vi "remove_instance.vi"(6 "id (unnamed)":string, 8 "error in (no error)":errorcluster, 9 "Object Instance":refnum<data-value>, 10 "Base Class (LabVIEW Object)":refnum<class>, 11 "Mapped Lookup in":refnum<class "Mapped Lookup.lvclass">) -> (0 "error out":errorcluster, 1 "removed?":bool, 3 "Mapped Lookup out":refnum<class "Mapped Lookup.lvclass">)   [LabVIEW 2019, in "Lookup API.lvlib" / "Mapped Lookup.lvclass"]
uses:
  Mapped Lookup.lvclass
  Mapped Lookup.lvclass/Mapped Lookup.ctl
  <vilib>/Utility/miscctls.llb/LVMapReplaceAction.ctl
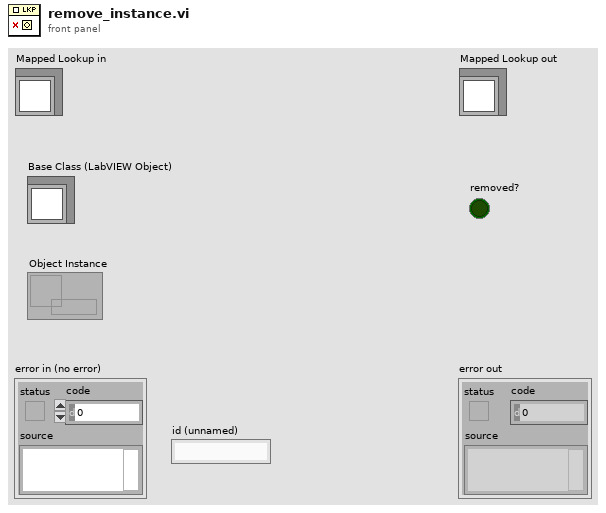
[diagram p1: front panel]
types:
  T1 = typedef "LVMapReplaceAction.ctl" = enum32{"Modify Entry only if found", "Add or Modify Entry", "Delete Entry"}
  T2 = map{string, cluster{"instances":refnum<data-value>, "events":refnum<data-value>}}
  T3 = cluster{"instances":refnum<data-value>, "events":refnum<data-value>}
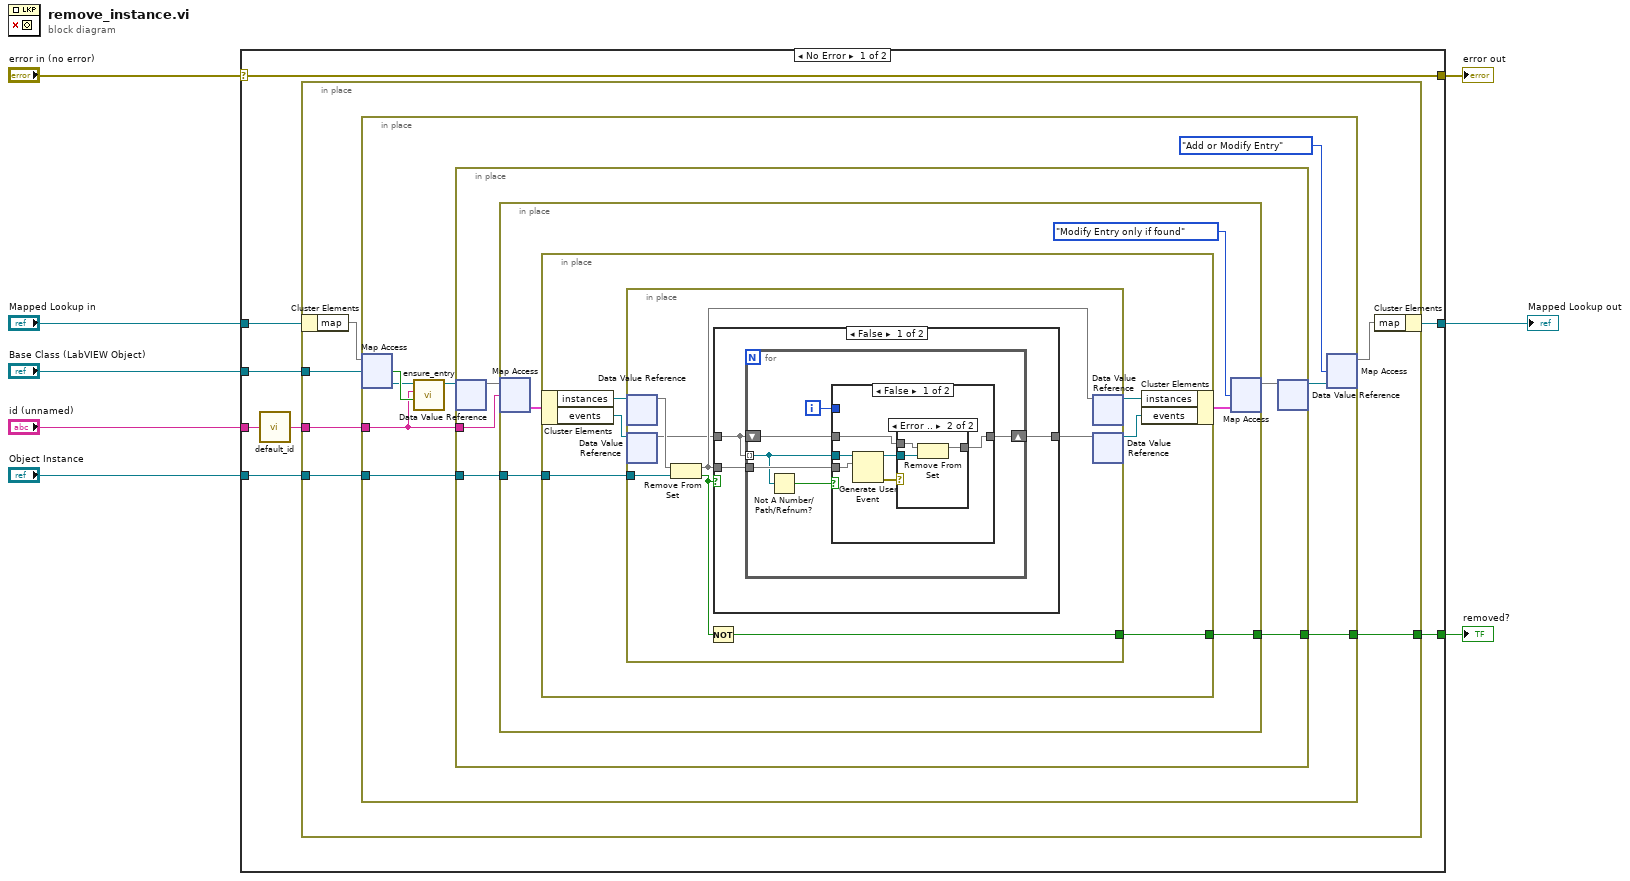
[diagram p0: block diagram]
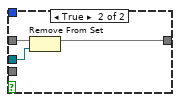
[diagram p3: hidden frame]
diagram:
  n1 = case shown="No Error" "error in (no error)" {
    selector: "error in (no error)" -> [w16 w78]
    tunnel: [w16 w78] -> w5
    tunnel: [w10 w77] -> w6
    tunnel: "Mapped Lookup in" -> [w15 w77]
    tunnel: "Base Class (LabVIEW Object)" -> [w14 _]
    tunnel: "id (unnamed)" -> [w13 _]
    tunnel: "Object Instance" -> [w11 _]
    tunnel: [w9 _] -> w2
    frame No Error {
      n2 = call "default_id.vi"("id (unnamed)"=w13) -> ("String"=w12:string)
      n3 = in-place {
        in-place-border: w14 -> [w18]
        in-place-border: w12 -> [w22]
        in-place-border: w11 -> [w21]
        in-place-border: [w17] -> w9
        n4 = in-place-cluster #1(w15) -> ("map"=w20:map{refnum<class>, refnum<data-value>})
        n5 = in-place {
          in-place-border: w22 -> [w25]
          in-place-border: w21 -> [w28]
          in-place-border: [w23] -> w17
          n6 = in-place-map #2(w20, w18) -> (w27:refnum<data-value>, w29:bool)  [unwired: 1 in]
          n7 = call "ensure_entry.vi"("not found?"=w29, "id"=w25, "named entries in"=w27) -> ("named entries out"=w26:refnum<data-value>)  [unwired: 8 in]
          n8 = in-place {
            in-place-border: w28 -> [w35]
            in-place-border: w25 -> [w33]
            in-place-border: [w31] -> w23
            n9 = in-place-dvr #3(w26) -> (w34:T2)  [unwired: 1 out]
            n10 = in-place {
              in-place-border: w35 -> [w40]
              in-place-border: [w36] -> w31
              n11 = in-place-map #4(w34, w33) -> (w39:T3)  [unwired: 1 in, 1 out]
              n12 = in-place {
                in-place-border: w40 -> [w46]
                in-place-border: [w41] -> w36
                n13 = in-place-cluster #5(w39) -> ("instances"=w45:refnum<data-value>, "events"=w43:refnum<data-value>)
                n14 = in-place {
                  in-place-border: w46 -> [w52]
                  in-place-border: [w48] -> w41
                  n15 = in-place-dvr #6(w45) -> (w53:set{refnum<data-value>})  [unwired: 1 out]
                  n16 = in-place-dvr #7(w43) -> (w50:set{refnum<user-event>})  [unwired: 1 out]
                  n17 = Remove From Set(10:w52, 11:w53) -> (2:w47:bool, 3:w51:set{refnum<data-value>})
                  n18 = Not(x=w47) -> (.not. x?=w48:bool)
                  n19 = case shown="False" w47 {
                    tunnel: w51 -> [w56 _]
                    tunnel: w50 -> [w55 w76]
                    tunnel: [w54 w76] -> w49
                    frame False {
                      n20 = for {
                        tunnel: w56 -> [w62]
                        tunnel: w55 -> [w61] mode=indexing
                        shift-right: [w57] -> w54
                        shift-left: w55 -> [w58]
                        i -> [w59]
                        n21 = Not A Number/Path/Refnum?(number/path/refnum=w61) -> (NaN/Path/Refnum?=w60:bool)
                        n22 = case shown="False" w60 {
                          tunnel: w62 -> [w68 _]
                          tunnel: w61 -> [w67 w74]
                          tunnel: w59 -> [_ _]
                          tunnel: w58 -> [w65 w75]
                          tunnel: [w64 w73] -> w57
                          frame False {
                            n23 = Generate User Event(user event=w67, event data cluster=w68) -> (user event out=w63:refnum<user-event>, error out=w66:errorcluster)  [unwired: 2 in]
                            n24 = case shown="Error .." w66 {
                              tunnel: w65 -> [w69 w72]
                              tunnel: [w69 w71] -> w64
                              tunnel: w63 -> [_ w70]
                              frame No Error {
                              }
                              frame Error {
                                n25 = Remove From Set(10:w70, 11:w72) -> (3:w71:set{refnum<user-event>})  [unwired: 1 out]
                              }
                            }
                          }
                          frame True {
                            n26 = Remove From Set(10:w74, 11:w75) -> (3:w73:set{refnum<user-event>})  [unwired: 1 out]
                          }
                        }
                      }
                    }
                    frame True {
                    }
                  }
                  n27 = in-place-dvr #6(w51) -> (w44:refnum<data-value>)  [unwired: 1 out]
                  n28 = in-place-dvr #7(w49) -> (w42:refnum<data-value>)  [unwired: 1 out]
                }
                n29 = in-place-cluster #5("instances"=w44, "events"=w42) -> (w38:T3)
              }
              n30 = in-place-map #4(w38, LVMapReplaceAction."Modify Entry only if found" ("action")) -> (w32:T2)  [unwired: 2 out]
            }
            n31 = in-place-dvr #3(w32) -> (w24:refnum<data-value>)  [unwired: 1 out]
          }
          n32 = in-place-map #2(w24, LVMapReplaceAction."Add or Modify Entry" ("action")) -> (w19:map{refnum<class>, refnum<data-value>})  [unwired: 2 out]
        }
        n33 = in-place-cluster #1("map"=w19) -> (w10:refnum<class "Mapped Lookup.lvclass">)
      }
    }
    frame Error {
    }
  }
  "error out" <- w5
  "Mapped Lookup out" <- w6
  "removed?" <- w2
